vi "Na-DAS_and_MAGIC_Pressures.vi"() -> (0 "DAQ Error":errorcluster)   [LabVIEW 2017]
doc: "Use this plug-in with the Nathan 7609 data acquisition system"
uses:
  MAGIC_Pressures/ctls/Cmd.ctl
  Globals/Meas_global.vi
  PWA/PWAtasksGLOBAL.vi
  Globals/Extra_Commands_Global.vi
  Globals/Dynamic_call_global.ph.vi
  Globals/Trav_pos_global.vi
panel:
  in  "Board 2 COM port":refnum<visa-resource-name>="COM31"
  in  "Pressure data rate (Hz)":u8(ring)=17 items=["1", "2", "4", "5", "8", "10", "16", "20", "25", "32", "40", "50", "64", "80", "100", "125", "160", "200", "250", "320", "400", "500", "625", "800", "1000"]
  in  "Board 1 COM port":refnum<visa-resource-name>="COM30"
  in  "Minimum timeout (ms)":u32=15000
  in  "Input voltage range (V)":u8(ring)=1 items=["-5... +5 V", "-10... +10 V"]
  out "Config read-back ok":bool
  out "Overruns":u32
  # "PN 25/11/2014, 19/12/2014, 15/02/2015 (channels in any order), 17/08/2015 (stop ack mod), 23/08/2015 (timeout mod for SW vs HW triggering), 03/09/2017 (rising and falling edge options for HW triggering)"
  # "Do not close this window between blocks"
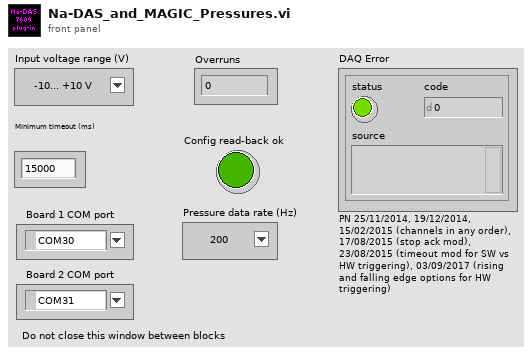
[diagram p1: front panel]
types:
  T1 = typedef "Ch_and_Spans.ctl" = cluster{"Sync Delay (ms)":dbl, "Ch No":i16, "Var name":string, "Use Latest Calib":bool, "Device ID":string}
  T2 = typedef "LDA_Setup.ctl" = cluster{"dimensions":enum16{"1D", "2D"}, "Analogue Freq Multiplier":dbl}
  T3 = typedef "Traverse_cluster.ctl" = cluster{"Start X":sgl, "Start Y":sgl, "Start Z":sgl, "End X":sgl, "End Y":sgl, "End Z":sgl, "No. of pts.":i32, "Spacing":T4, "Filename":path, "Tunnel Speed":dbl, "Averaging time (min)":dbl, "Extra Commands":string, "Carrier_1 Q (l/min)":dbl, "Carrier_2 Q (l/min)":dbl, "Trace Gas Concentration (%)":dbl, "Specific Arguments":string, "Comments":string, "Row No":i32, "Row Type Selector":T5, "Completion time":string, "Row Duration (mins)":dbl, "No. of Valid pts.":i32, "Meas Setup File":string}
  T4 = typedef "Spacing.ctl" = enum16{"Linear", "Log", "Gauss", "Specified", "N/A"}
  T5 = typedef "Multi_run_mode.ctl" = enum16{"Move Traverse Only", "Set Tunnel Speed Only", "Set Source Only", "Set Measurement Conditions", "Single Measurement", "Vertical Profile", "Lateral Profile", "Longitudinal Profile", "Explore Volume", "Multi-Axis Profile", "Auto Calibrate", "Meas Fast FID Bkgnd", "Check Beam Power", "Scanning Valve Measurement", "Run VI Named:", "Set ADAM Ch", "Wait (minutes)", "Send Message", "Synchronize With:", "Fall Back to this Row", "Turn Off Row Repeating", "Blank Row", "Traverse 3D Volume"}
  T6 = typedef "Trigger_Mode.ctl" = enum16{"Free Running", "Start on Trigger", "Trigger Every Block", "Trigger Every Sample"}
  T7 = typedef "Cmd.ctl" = string
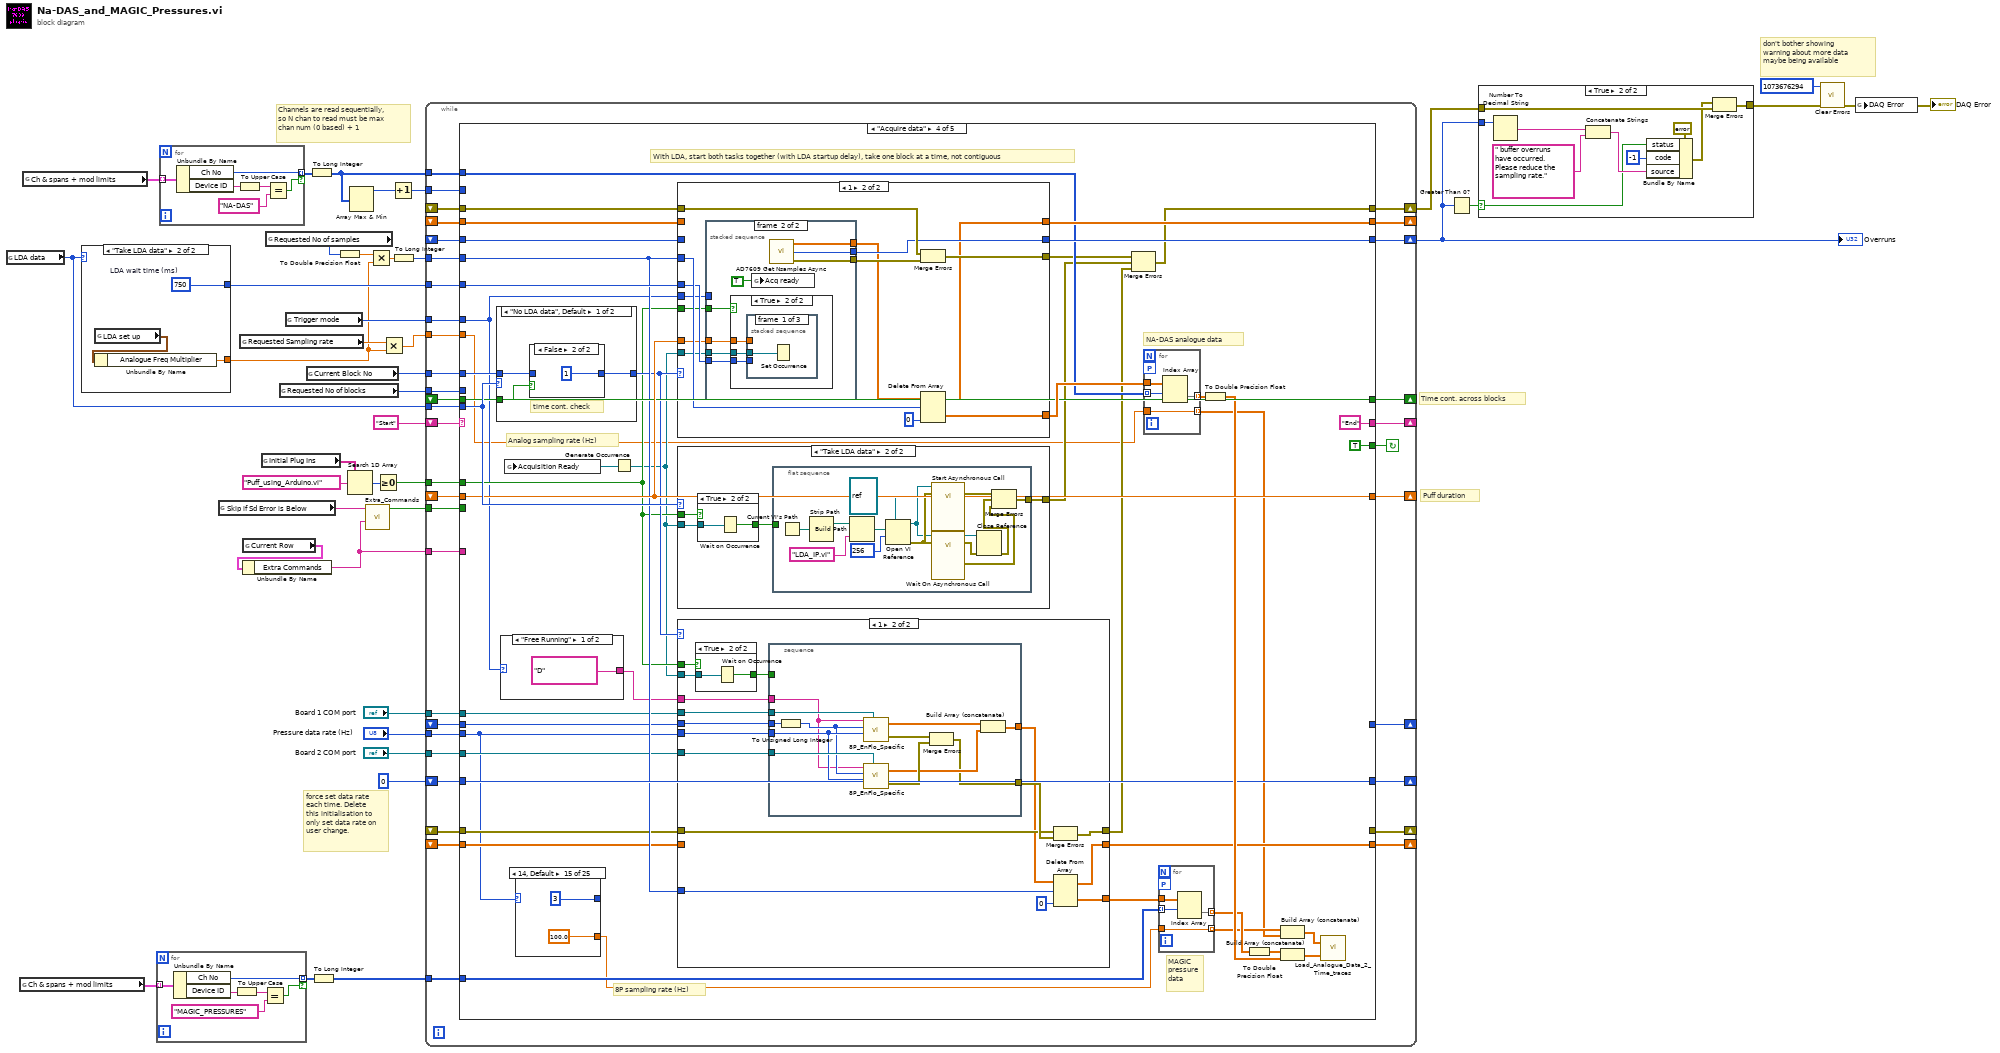
[diagram p0: block diagram]
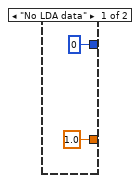
[diagram p2: hidden frame]
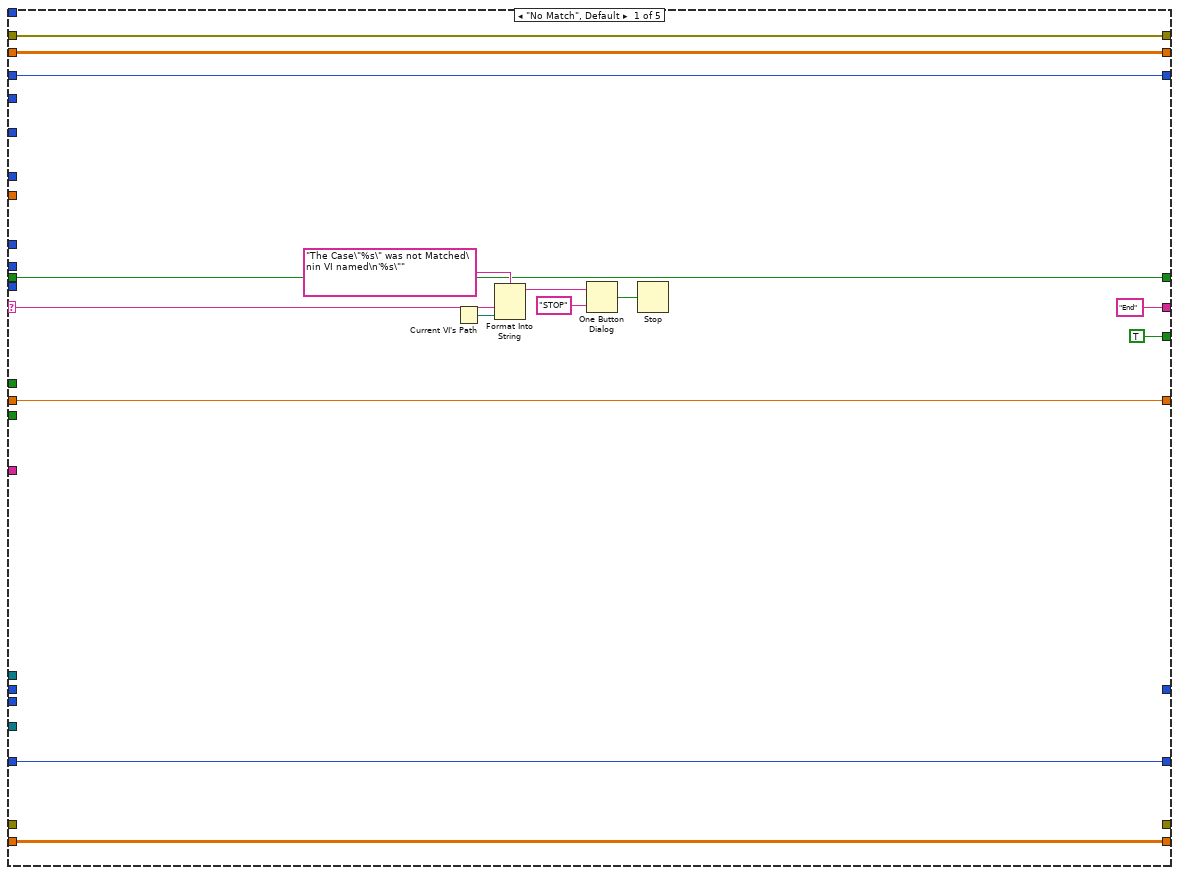
[diagram p3: hidden frame]
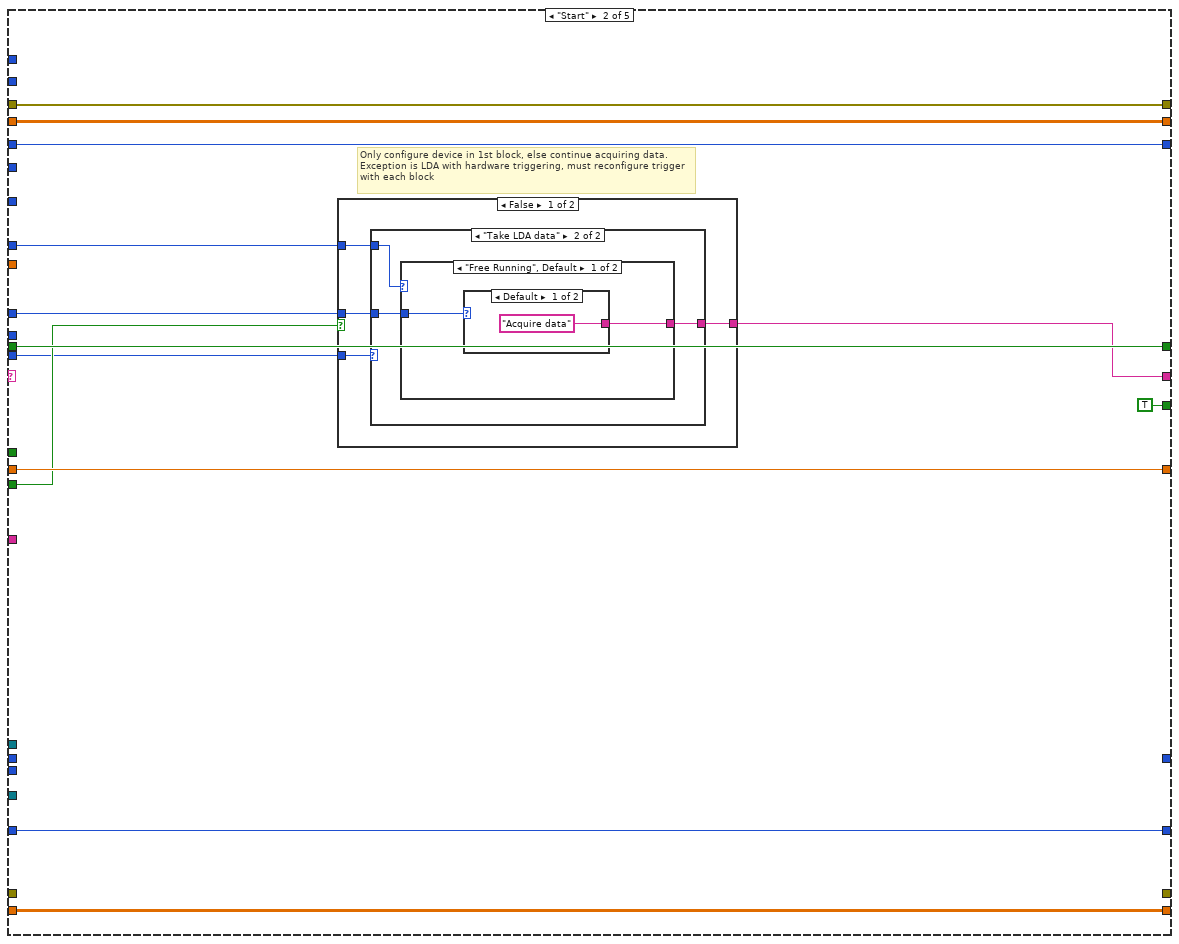
[diagram p4: hidden frame]
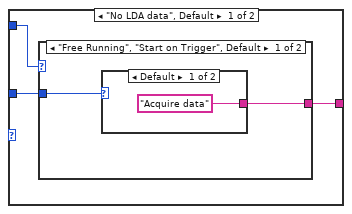
[diagram p5: hidden frame]
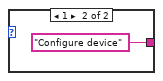
[diagram p6: hidden frame]
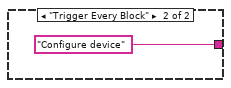
[diagram p7: hidden frame]
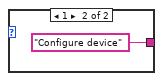
[diagram p8: hidden frame]
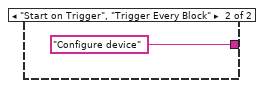
[diagram p9: hidden frame]
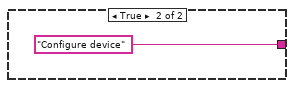
[diagram p10: hidden frame]
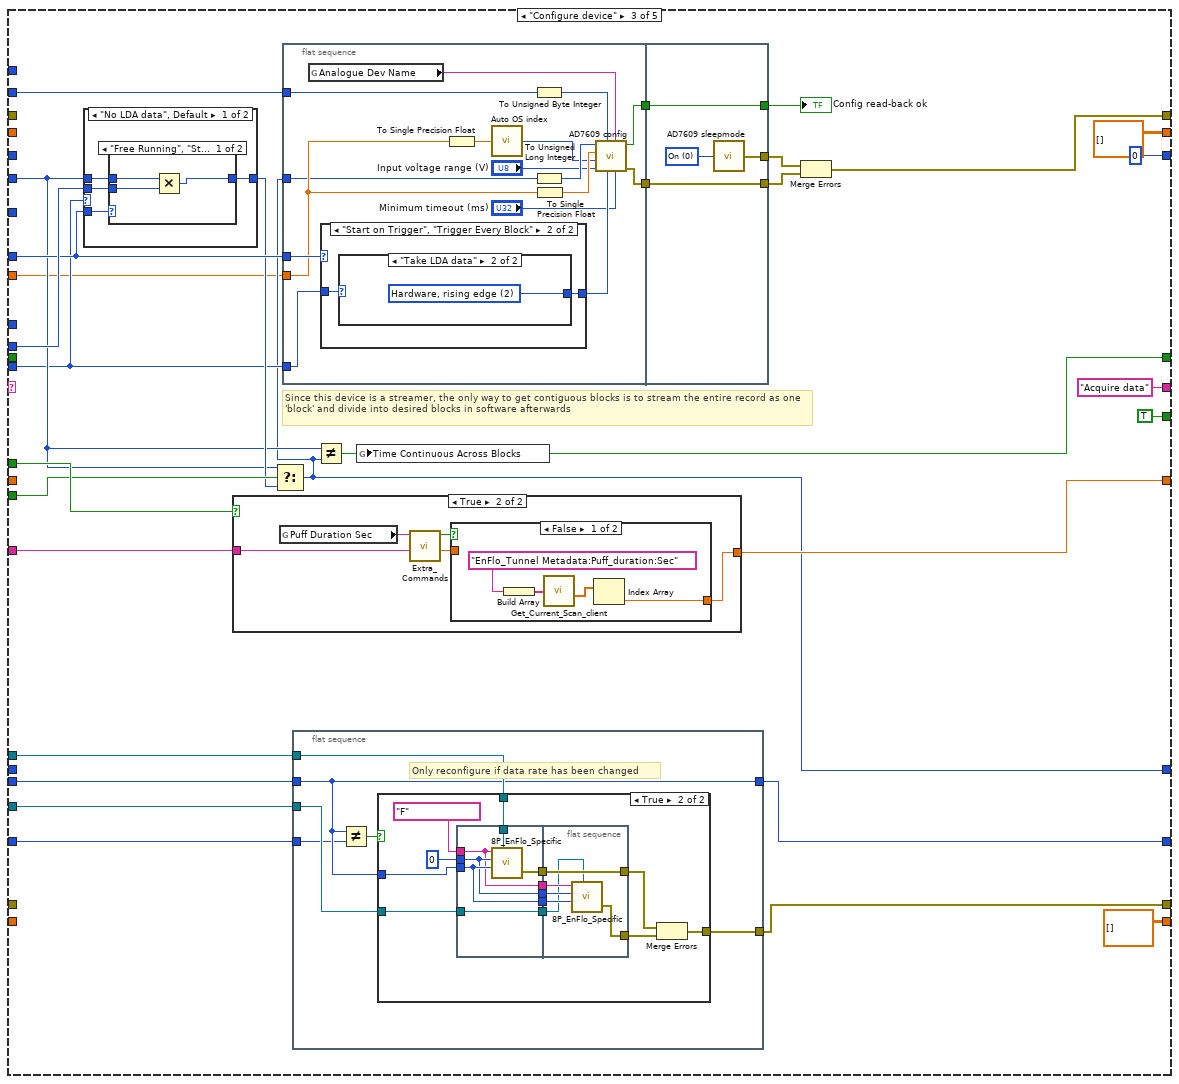
[diagram p11: hidden frame]
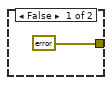
[diagram p12: hidden frame]
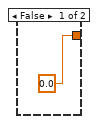
[diagram p13: hidden frame]
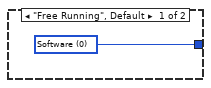
[diagram p17: hidden frame]
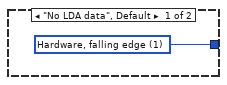
[diagram p18: hidden frame]
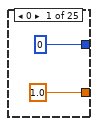
[diagram p19: hidden frame]
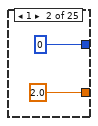
[diagram p20: hidden frame]
diagram:
  # "force set data rate each time. Delete this initialisation to only set data rate on user change."
  # "don't bother showing warning about more data maybe being available"
  # "Time cont. across blocks"
  # "Puff duration"
  # "Channels are read sequentially, so N chan to read must be max chan num (0 based) + 1"
  n1 = global read "Meas_global.vi" "LDA data"() -> (w34:enum16{"No LDA data", "Take LDA data"})
  n2 = global read "Meas_global.vi" "Ch & spans + mod limits"() -> (w3:T1[])
  n3 = global read "Meas_global.vi" "Ch & spans + mod limits"() -> (w20:T1[])
  n4 = case shown="\"Take LDA data\"" w34 {
    tunnel: [1.0 ("Analogue Freq Multiplier") w43] -> w25
    tunnel: [u32 0 ("LDA wait time (ms)") w42] -> w29
    frame "No LDA data" {
    }
    frame "Take LDA data" {
      w42 = u32 750  # LDA wait time (ms)
      n5 = global read "Meas_global.vi" "LDA set up"() -> (w44:T2)
      n6 = Unbundle By Name(w44) -> ("Analogue Freq Multiplier"=w43:dbl)
    }
  }
  n7 = for {
    tunnel: w3 -> [w50] mode=indexing
    tunnel: [w49] -> w4 mode=indexing if=w45
    n8 = Unbundle By Name(w50) -> ("Ch No"=w49:i16, "Device ID"=w48:string)
    n9 = To Upper Case(1:w48) -> (0:w47:string)
    n10 = Equal?(x=w47, y="MAGIC_PRESSURES") -> (x = y?=w45:bool)
  }
  n11 = for {
    tunnel: w20 -> [w56] mode=indexing
    tunnel: [w55] -> w19 mode=indexing if=w51
    n12 = Unbundle By Name(w56) -> ("Ch No"=w55:i16, "Device ID"=w54:string)
    n13 = To Upper Case(1:w54) -> (0:w53:string)
    n14 = Equal?(x=w53, y="NA-DAS") -> (x = y?=w51:bool)
  }
  n15 = global read "Extra_Commands_Global.vi" "Skip if Sd Error is Below"() -> (w15:string)
  n16 = global read "Meas_global.vi" "Requested Sampling rate"() -> (w35:dbl)
  n17 = global read "Trav_pos_global.vi" "Current Row"() -> (w16:T3)
  n18 = Unbundle By Name(w16) -> ("Extra Commands"=w14:string)
  n19 = global read "Dynamic_call_global.ph.vi" "Initial Plug Ins"() -> (w31:string[])
  n20 = global read "Meas_global.vi" "Requested No of samples"() -> (w26:i32)
  n21 = global read "Meas_global.vi" "Requested No of blocks"() -> (w22:i32)
  n22 = global read "Meas_global.vi" "Trigger mode"() -> (w38:T6)
  n23 = global read "Meas_global.vi" "Current Block No"() -> (w37:i32)
  n24 = To Long Integer(number=w19) -> (32bit integer=w1:i32[])
  n25 = To Long Integer(number=w4) -> (32bit integer=w2:i32[])
  n26 = To Double Precision Float(number=w26) -> (double precision float=w24:dbl)
  n27 = Search 1D Array(1D array=w31, element="Puff_using_Arduino.vi") -> (index of element=w33:i32)  [unwired: 1 in]
  n28 = Array Max & Min(array=w1) -> (max value=w18:i32)  [unwired: 3 out]
  n29 = call "Extra_Commands.vi"("String to Search"=w14, "Command"=w15) -> ("Command Found"=w13:bool)  [unwired: 2 in, 3 out]
  n30 = Multiply(x=w24, y=w25) -> (x*y=w23:dbl)
  n31 = Greater Or Equal To 0?(x=w33) -> (x >= 0?=w30:bool)
  n32 = Multiply(x=w35, y=w25) -> (x*y=w36:dbl)
  n33 = Increment(x=w18) -> (x+1=w17:i32)
  n34 = To Long Integer(number=w23) -> (32bit integer=w21:i32)
  n35 = while {
    shift-left: "Start" -> [w93]
    shift-right: [w79] -> _
    tunnel: w36 -> [w92]
    tunnel: w21 -> [w91]
    tunnel: w37 -> [w90]
    tunnel: w38 -> [w88]
    tunnel: w34 -> [w87]
    tunnel: w22 -> [w86]
    shift-right: [w84] -> w28
    shift-left: _ -> [w85]
    shift-right: [w83] -> _
    shift-left: _ -> [w82]
    shift-right: [w81] -> w11
    shift-left: _ -> [w80]
    tunnel: w29 -> [w78]
    tunnel: w30 -> [w77]
    shift-right: [w76] -> _
    shift-left: _ -> [w75]
    tunnel: w17 -> [w74]
    tunnel: w14 -> [w73]
    tunnel: w13 -> [w72]
    shift-right: [w71] -> _
    shift-left: _ -> [w70]
    tunnel: "Board 1 COM port" -> [w69]
    tunnel: "Pressure data rate (Hz)" -> [w68]
    tunnel: "Board 2 COM port" -> [w67]
    shift-right: [w65] -> _
    shift-left: u8 0 ("Pressure data rate (Hz)") -> [w66]
    shift-right: [w64] -> _
    shift-left: _ -> [w61]
    shift-right: [w62] -> _
    shift-left: _ -> [w63]
    shift-right: [w60] -> _
    shift-left: _ -> [w59]
    tunnel: w2 -> [w58]
    tunnel: w1 -> [w57]
    stop <- w89 continue-if-true
    n36 = case shown="\"Acquire data\"" w93 {
      selector: w93 -> [w101 _ _ _ _]
      tunnel: ["End" w111 "Acquire data" ("f") "End" "End" ("f")] -> w79
      tunnel: w92 -> [_ _ w143 w252 _]
      tunnel: w91 -> [_ _ w154 w272 _]
      tunnel: w90 -> [_ w114 _ w286 w467]
      tunnel: [TRUE TRUE TRUE TRUE FALSE] -> w89
      tunnel: w88 -> [_ w113 w161 w258 _]
      tunnel: w87 -> [_ w112 w152 w284 _]
      tunnel: w86 -> [_ _ w170 _ w468]
      tunnel: w85 -> [w100 w120 _ w291 w465]
      tunnel: [w100 w120 w171 w276 w464] -> w84
      tunnel: [w99 w119 sgl[][] [] ("Channel volts") w287 w463] -> w83
      tunnel: w82 -> [w99 w119 _ w288 w463]
      tunnel: [w98 w118 u32 0 ("Overruns") w290 w462] -> w81
      tunnel: w80 -> [w98 w118 _ w289 w462]
      tunnel: w78 -> [_ _ _ w285 _]
      tunnel: w77 -> [_ _ w160 w261 _]
      tunnel: [w97 w117 w159 w283 w461] -> w76
      tunnel: w75 -> [w97 w117 _ w283 w461]
      tunnel: w57 -> [_ _ _ w281 _]
      tunnel: w74 -> [_ _ w158 _ _]
      tunnel: w73 -> [_ _ w157 _ _]
      tunnel: w72 -> [_ w115 w156 _ _]
      tunnel: [w96 w116 w153 w279 w460] -> w71
      tunnel: w70 -> [w96 w116 _ w279 w460]
      tunnel: w69 -> [_ _ w151 w268 _]
      tunnel: w68 -> [_ _ w149 w251 _]
      tunnel: w67 -> [_ _ w150 w269 _]
      tunnel: w66 -> [w95 w110 w148 w273 w459]
      tunnel: [w95 w110 w147 w273 w459] -> w65
      tunnel: [_ _ w146 _ _] -> w64
      tunnel: w63 -> [_ _ _ w270 _]
      tunnel: [_ _ w145 _ _] -> w62
      tunnel: w61 -> [_ _ _ w267 _]
      tunnel: [w94 w109 sgl[][] [] ("Channel volts") w266 w458] -> w60
      tunnel: w59 -> [w94 w109 _ w263 w458]
      tunnel: w58 -> [_ _ _ w253 _]
      frame "No Match", Default {
        n37 = Current VI's Path() -> (path=w104:path)
        n38 = Format Into String(format string="The Case\"%s\" was not Matched\nin VI named\n'%s\"" ("Format String"), w101, w104) -> (resulting string=w107:string)  [unwired: 2 in, 1 out]
        n39 = One Button Dialog(message=w107, button name ("OK")="STOP") -> (true=w105:bool)
        n40 = Stop(stop? (T)=w105) -> ()
      }
      frame "Start" {
        # "Only configure device in 1st block, else continue acquiring data. Exception is LDA with hardware triggering, must reconfigure trigger with each block"
        n41 = case shown="False" w115 {
          tunnel: w114 -> [w125 _]
          tunnel: [w124 "Configure device" ("f")] -> w111
          tunnel: w112 -> [w123 _]
          tunnel: w113 -> [w122 _]
          frame False {
            n42 = case shown="\"Take LDA data\"" w123 {
              tunnel: w125 -> [w128 w134]
              tunnel: [w127 w135] -> w124
              tunnel: w122 -> [w126 w136]
              frame "No LDA data", Default {
                n43 = case shown="\"Free Running\", \"Start on Trigger\", Default" w126 {
                  tunnel: w128 -> [w130 _]
                  tunnel: [w129 "Configure device" ("f")] -> w127
                  frame "Free Running", "Start on Trigger", Default {
                    n44 = case shown="Default" w130 {
                      tunnel: ["Acquire data" ("f") "Configure device" ("f")] -> w129
                      frame Default {
                      }
                      frame 1 {
                      }
                    }
                  }
                  frame "Trigger Every Block" {
                  }
                }
              }
              frame "Take LDA data" {
                n45 = case shown="\"Free Running\", Default" w136 {
                  tunnel: [w138 "Configure device" ("f")] -> w135
                  tunnel: w134 -> [w137 _]
                  frame "Free Running", Default {
                    n46 = case shown="Default" w137 {
                      tunnel: ["Acquire data" ("f") "Configure device" ("f")] -> w138
                      frame Default {
                      }
                      frame 1 {
                      }
                    }
                  }
                  frame "Start on Trigger", "Trigger Every Block" {
                  }
                }
              }
            }
          }
          frame True {
          }
        }
      }
      frame "Configure device" {
        # "Since this device is a streamer, the only way to get contiguous blocks is to stream the entire record as one 'block' and divide into desired blocks in software afterwards"
        n47 = case shown="\"No LDA data\", Default" w152 {
          tunnel: [w217 w224] -> w155
          tunnel: w154 -> [w219 w224]
          tunnel: w170 -> [w218 _]
          tunnel: w161 -> [w216 _]
          frame "No LDA data", Default {
            n48 = case shown="\"Free Running\", \"Start on Trigger\"" w216 {
              tunnel: w219 -> [w222 w223]
              tunnel: w218 -> [w221 _]
              tunnel: [w220 w223] -> w217
              frame "Free Running", "Start on Trigger" {
                n49 = Multiply(x=w222, y=w221) -> (x*y=w220:i32)
              }
              frame "Trigger Every Block", Default {
              }
            }
          }
          frame "Take LDA data" {
          }
        }
        n50 = case shown="True" w160 {
          tunnel: [0.0 w210] -> w159
          tunnel: w157 -> [_ w206]
          frame False {
          }
          frame True {
            n51 = global read "Extra_Commands_Global.vi" "Puff Duration Sec"() -> (w209:string)
            n52 = call "Extra_Commands.vi"("String to Search"=w206, "Command"=w209) -> ("Numeric Value"=w207:dbl, "Command Found"=w208:bool)  [unwired: 2 in, 2 out]
            n53 = case shown="False" w208 {
              tunnel: [w211 w215] -> w210
              tunnel: w207 -> [_ w215]
              frame False {
                n54 = Build Array("EnFlo_Tunnel Metadata:Puff_duration:Sec") -> (w213:string[])
                n55 = call "Get_Current_Scan_client.vi"("ADAM Ch Names"=w213) -> ("Numerical Values"=w214:dbl[])  [unwired: 1 in, 2 out]
                n56 = Index Array(array=w214) -> (element=w211:dbl)  [unwired: 1 in]
              }
              frame True {
              }
            }
          }
        }
        n57 = Select(t=w154, s=w156, f=w155) -> (s? t:f=w146:i32)
        n58 = flat-sequence {
          tunnel: w146 -> [w225]
          tunnel: w143 -> [w231]
          tunnel: w161 -> [w240]
          tunnel: [w234] -> w169
          tunnel: [w233] -> w168
          tunnel: w158 -> [w228]
          tunnel: w152 -> [w226]
          tunnel: [w248] -> w165
          tunnel: w169 -> [w248]
          tunnel: [w247] -> w167
          tunnel: w168 -> [w247]
          tunnel: [w246] -> w166
          frame #0 {
            n59 = global read "PWAtasksGLOBAL.vi" "Analogue Dev Name"() -> (w239:string)
            n60 = case shown="\"Start on Trigger\", \"Trigger Every Block\"" w240 {
              tunnel: [w241 w243] -> w236
              tunnel: w226 -> [_ w242]
              frame "Free Running", Default {
                w241 = u8 0 items=["Software", "Hardware, falling edge", "Hardware, rising edge"] ("Triggering mode")
              }
              frame "Start on Trigger", "Trigger Every Block" {
                n61 = case shown="\"Take LDA data\"" w242 {
                  tunnel: [w244 w245] -> w243
                  frame "No LDA data", Default {
                    w244 = u8 1 items=["Software", "Hardware, falling edge", "Hardware, rising edge"] ("Triggering mode")
                  }
                  frame "Take LDA data" {
                    w245 = u8 2 items=["Software", "Hardware, falling edge", "Hardware, rising edge"] ("Triggering mode")
                  }
                }
              }
            }
            n62 = To Single Precision Float(number=w231) -> (single precision float=w229:sgl)
            n63 = call "Auto OS index.vi"("Sampling rate"=w229) -> ("OS index"=w230:u8)
            n64 = To Unsigned Byte Integer(number=w228) -> (unsigned 8bit integer=w235:u8)
            n65 = To Unsigned Long Integer(number=w225) -> (unsigned 32bit integer=w238:u32)
            n66 = To Single Precision Float(number=w231) -> (single precision float=w237:sgl)
            n67 = call "AD7609 config.vi"("Timeout for software trig. mode (ms)"="Minimum timeout (ms)", "Device serial port"=w239, "Triggering mode"=w236, "N channels to read"=w235, "Input voltage range (V)"="Input voltage range (V)", "Oversampling ratio"=w230, "Sampling rate (Hz)"=w237, "Number of samples"=w238) -> ("Config error out"=w233:errorcluster, "Config read-back ok"=w234:bool)  [unwired: 2 in]
          }
          frame #1 {
            w249 = u8 0 items=["On", "Standby", "Shutdown"] ("Sleep state")
            n68 = call "AD7609 sleepmode.vi"("Sleep state"=w249) -> ("Sleep error out"=w246:errorcluster)
          }
        }
        n69 = flat-sequence {
          tunnel: [w178] -> w145
          tunnel: w151 -> [w177]
          tunnel: w150 -> [w176]
          tunnel: w149 -> [w174]
          tunnel: [w174] -> w147
          tunnel: w148 -> [w173]
          frame #0 {
            # "Only reconfigure if data rate has been changed"
            n70 = Not Equal?(x=w174, y=w173) -> (x != y?=w175:bool)
            n71 = case shown="True" w175 {
              tunnel: [errorcluster {"status"=FALSE, "code"=0, "source"=""} ("error IO") w191] -> w178
              tunnel: w177 -> [_ w190]
              tunnel: w176 -> [_ w180]
              tunnel: w174 -> [_ w187]
              frame False {
              }
              frame True {
                n72 = flat-sequence {
                  tunnel: w190 -> [w194]
                  tunnel: T7 "F" ("Command") -> [w195]
                  tunnel: u32 0 ("N samples") -> [w196]
                  tunnel: w187 -> [w197]
                  tunnel: [w198] -> w185
                  tunnel: [w197] -> w184
                  tunnel: [w196] -> w183
                  tunnel: [w195] -> w182
                  tunnel: [w193] -> w181
                  tunnel: w180 -> [w193]
                  tunnel: [w204] -> w192
                  tunnel: [w200] -> w186
                  tunnel: w181 -> [w199]
                  tunnel: w182 -> [w201]
                  tunnel: w183 -> [w202]
                  tunnel: w184 -> [w203]
                  tunnel: w185 -> [w204]
                  frame #0 {
                    n73 = call "8P_EnFlo_Specific.vi"("COM port"=w194, "Data rate (Hz)"=w197, "N samples"=w196, "Command"=w195) -> ("Error"=w198:errorcluster)  [unwired: 2 in, 1 out]
                  }
                  frame #1 {
                    n74 = call "8P_EnFlo_Specific.vi"("COM port"=w199, "Data rate (Hz)"=w203, "N samples"=w202, "Command"=w201) -> ("Error"=w200:errorcluster)  [unwired: 2 in, 1 out]
                  }
                }
                n75 = Merge Errors(w192, w186) -> (w191:errorcluster)
              }
            }
          }
        }
        n76 = Not Equal?(x=w154, y=w146) -> (x != y?=w153:bool)
        n77 = global write "Meas_global.vi" "Time Continuous Across Blocks"(w153) -> ()
        n78 = Merge Errors(w166, w167) -> (w171:errorcluster)
        "Config read-back ok" <- w165
      }
      frame "Acquire data" {
        # "Analog sampling rate (Hz)"
        # "8P sampling rate (Hz)"
        # "MAGIC\npressure\ndata"
        # "NA-DAS analogue data"
        # "With LDA, start both tasks together (with LDA startup delay), take one block at a time, not contiguous"
        n79 = case shown="\"No LDA data\", Default" w284 {
          tunnel: w286 -> [w414 _]
          tunnel: [w415 1 ("Current Block No")] -> w271
          tunnel: w279 -> [w413 _]
          frame "No LDA data", Default {
            # "time cont. check"
            n80 = case shown="False" w413 {
              tunnel: [w416 1 ("Current Block No")] -> w415
              tunnel: w414 -> [w416 _]
              frame True {
              }
              frame False {
              }
            }
          }
          frame "Take LDA data" {
          }
        }
        n81 = case shown="\"Free Running\"" w258 {
          tunnel: [T7 "D" ("Combo Box") T7 "T" ("Combo Box")] -> w257
          frame "Free Running" {
          }
          frame Default {
          }
        }
        n82 = case shown="14, Default" w251 {
          tunnel: [1.0 2.0 4.0 5.0 8.0 10.0 16.0 20.0 25.0 32.0 40.0 50.0 64.0 80.0 100.0 125.0 160.0 200.0 250.0 320.0 400.0 500.0 625.0 800.0 1000.0] -> w250
          tunnel: [u8 0 u8 0 u8 0 u8 0 u8 0 u8 0 u8 0 u8 0 u8 1 u8 1 u8 1 u8 2 u8 2 u8 2 u8 3 u8 3 u8 3 u8 4 u8 4 u8 4 u8 5 u8 5 u8 6 u8 6 u8 6] -> _
          frame 0 {
          }
          frame 1 {
          }
          frame 2 {
          }
          frame 3 {
          }
          frame 4 {
          }
          frame 5 {
          }
          frame 6 {
          }
          frame 7 {
          }
          frame 8 {
          }
          frame 9 {
          }
          frame 10 {
          }
          frame 11 {
          }
          frame 12 {
          }
          frame 13 {
          }
          frame 14, Default {
          }
          frame 15 {
          }
          frame 16 {
          }
          frame 17 {
          }
          frame 18 {
          }
          frame 19 {
          }
          frame 20 {
          }
          frame 21 {
          }
          frame 22 {
          }
          frame 23 {
          }
          frame 24 {
          }
        }
        n83 = Generate Occurrence() -> (w260:refnum<k4>)
        n84 = global write "Meas_global.vi" "Acquisition Ready"(w260) -> ()
        n85 = case shown="1" w271 {
          tunnel: w291 -> [w420 w438]
          tunnel: [w420 w437] -> w278
          tunnel: [w421 w436] -> w290
          tunnel: [w423 w433] -> w287
          tunnel: w272 -> [w422 w434]
          tunnel: w288 -> [w424 _]
          tunnel: w289 -> [w421 _]
          tunnel: [w419 w431] -> w282
          tunnel: w285 -> [_ w430]
          tunnel: w260 -> [_ w429]
          tunnel: w261 -> [_ w428]
          tunnel: w283 -> [_ w427]
          tunnel: w258 -> [_ w426]
          frame Default {
            # "First block gets ALL samples (N_blocks * samples per block). Output one block of samples and keep remainder for next block cycle."
            n86 = Delete From Array(array=w424, length=w422, index (col)=0 ("disabled index (col)")) -> (deleted portion=w419:sgl[][], array with subset deleted=w423:sgl[][])  [unwired: 1 in]
          }
          frame 1 {
            n87 = stacked-sequence {
              tunnel: [_ w449] -> w436
              tunnel: [_ w448] -> w435
              tunnel: [_ w447] -> w439
              tunnel: w429 -> [_ w446]
              tunnel: w430 -> [w441 w445]
              tunnel: w428 -> [_ w444]
              tunnel: w427 -> [_ w443]
              tunnel: w426 -> [w440 _]
              frame #0 {
                n88 = case shown="\"Free Running\"" w440 {
                  tunnel: w441 -> [w442 _]
                  frame "Free Running" {
                    n89 = Wait (ms)(milliseconds to wait=w442) -> ()  [unwired: 1 out]
                  }
                  frame Default {
                  }
                }
              }
              frame #1 {
                n90 = case shown="True" w444 {
                  tunnel: w446 -> [w451 w454]
                  tunnel: w443 -> [_ w453]
                  tunnel: w445 -> [_ w452]
                  frame False {
                    n91 = Set Occurrence(w451) -> ()
                  }
                  frame True {
                    n92 = stacked-sequence {
                      tunnel: w454 -> [w455 _ _]
                      tunnel: w453 -> [_ _ w457]
                      tunnel: w452 -> [_ w456 _]
                      frame #0 {
                        n93 = Set Occurrence(w455) -> ()
                      }
                      frame #1 {
                        n94 = Wait (ms)(milliseconds to wait=w456) -> ()  [unwired: 1 out]
                      }
                      frame #2 {
                        n95 = call "Puff_using_Arduino_oneshot.vi"("Puff_duration:Sec"=w457) -> ()  [unwired: 7 in]
                      }
                    }
                  }
                }
                n96 = global write "Meas_global.vi" "Acq ready"(TRUE ("Acq ready")) -> ()
                n97 = call "AD7609 Get Nsamples Async.vi"() -> ("Channel volts"=w448:sgl[][], "Overruns"=w449:u32, "Async error"=w447:errorcluster)  [unwired: 1 in]
              }
            }
            n98 = Merge Errors(w438, w439) -> (w437:errorcluster)
            n99 = Delete From Array(array=w435, length=w434, index (col)=0 ("disabled index (col)")) -> (deleted portion=w431:sgl[][], array with subset deleted=w433:sgl[][])  [unwired: 1 in]
          }
        }
        n100 = case shown="\"Take LDA data\"" w284 {
          tunnel: w261 -> [_ w392]
          tunnel: w260 -> [_ w394]
          tunnel: [errorcluster {"status"=FALSE, "code"=0, "source"=""} ("error IO") w393] -> w277
          frame "No LDA data", Default {
          }
          frame "Take LDA data" {
            n101 = case shown="True" w392 {
              tunnel: [FALSE ("timed out") w398] -> w395
              tunnel: w394 -> [_ w397]
              frame False {
              }
              frame True {
                n102 = Wait on Occurrence(2:w397) -> (0:w398:bool)  [unwired: 2 in]
              }
            }
            n103 = flat-sequence {
              tunnel: w395 -> [_]
              tunnel: [w400] -> w393
              frame #0 {
                n104 = Current VI's Path() -> (path=w410:path)
                n105 = Strip Path(path=w410) -> (stripped path=w409:path)  [unwired: 1 out]
                n106 = Build Path(base path=w409, name or relative path="LDA_IP.vi") -> (appended path=w411:path)
                n107 = Open VI Reference(type specifier VI Refnum (for type only)=refnum<vi> refnum, vi path=w411, options=256) -> (vi reference=w405:refnum<vi>, error out=w406:errorcluster)  [unwired: 3 in]
                n108 = call-by-ref "Start Asynchronous Call"(reference=w405, error in=w406) -> (error out=w402:errorcluster)  [unwired: 1 in, 2 out]
                n109 = call-by-ref "Wait On Asynchronous Call"(reference=w405, error in=w406) -> (reference out=w404:refnum<vi>, error out=w403:errorcluster, 0:"error out"=w399:errorcluster)  [unwired: 1 in]
                n110 = Close Reference(reference=w404, error in (no error)=w403) -> (error out=w401:errorcluster)
                n111 = Merge Errors(w402, w401, w399) -> (w400:errorcluster)
              }
            }
          }
        }
        n112 = case shown="1" w271 {
          tunnel: w270 -> [w351 w370]
          tunnel: [w351 w369] -> w262
          tunnel: [w353 w366] -> w266
          tunnel: w272 -> [w352 w367]
          tunnel: w263 -> [w354 _]
          tunnel: [w350 w364] -> w265
          tunnel: w268 -> [_ w363]
          tunnel: w269 -> [_ w362]
          tunnel: w251 -> [_ w361]
          tunnel: w267 -> [_ w360]
          tunnel: w261 -> [_ w358]
          tunnel: w260 -> [_ w357]
          tunnel: w257 -> [_ w356]
          frame Default {
            # "First block gets ALL samples (N_blocks * samples per block). Output one block of samples and keep remainder for next block cycle."
            n113 = Delete From Array(array=w354, length=w352, index (col)=0 ("disabled index (col)")) -> (deleted portion=w350:sgl[][], array with subset deleted=w353:sgl[][])  [unwired: 1 in]
          }
          frame 1 {
            n114 = case shown="True" w358 {
              tunnel: [FALSE ("timed out") w374] -> w359
              tunnel: w357 -> [_ w373]
              frame False {
              }
              frame True {
                n115 = Wait on Occurrence(2:w373) -> (0:w374:bool)  [unwired: 2 in]
              }
            }
            n116 = stacked-sequence {
              tunnel: [w378] -> w368
              tunnel: [w377] -> w371
              tunnel: w363 -> [w384]
              tunnel: w362 -> [w383]
              tunnel: w361 -> [w382]
              tunnel: w360 -> [w379]
              tunnel: w359 -> [_]
              tunnel: w356 -> [w375]
              frame #0 {
                n117 = To Unsigned Long Integer(number=w379) -> (unsigned 32bit integer=w376:u32)
                n118 = call "8P_EnFlo_Specific.vi"("COM port"=w384, "Data rate (Hz)"=w382, "N samples"=w376, "Command"=w375) -> ("Error"=w385:errorcluster, "All samples out"=w380:sgl[][])  [unwired: 2 in]
                n119 = call "8P_EnFlo_Specific.vi"("COM port"=w383, "Data rate (Hz)"=w382, "N samples"=w376, "Command"=w375) -> ("Error"=w386:errorcluster, "All samples out"=w381:sgl[][])  [unwired: 2 in]
                n120 = Merge Errors(w385, w386) -> (w377:errorcluster)
                n121 = Build Array (concatenate)(w380, w381) -> (w378:sgl[][])
              }
            }
            n122 = Merge Errors(w370, w371) -> (w369:errorcluster)
            n123 = Delete From Array(array=w368, length=w367, index (col)=0 ("disabled index (col)")) -> (deleted portion=w364:sgl[][], array with subset deleted=w366:sgl[][])  [unwired: 1 in]
          }
        }
        n124 = Merge Errors(w278, w277, w262) -> (w276:errorcluster)
        n125 = for {
          tunnel: w281 -> [w389] mode=indexing
          tunnel: [w388] -> w280 mode=indexing
          workers-P: _ -> [_]
          tunnel: w282 -> [w390]
          tunnel: [w387] -> w255 mode=indexing
          tunnel: w252 -> [w387]
          n126 = Index Array(array=w390, index (row)=w389) -> (element=w388:sgl[])  [unwired: 1 in]
        }
        n127 = for {
          tunnel: w253 -> [w348] mode=indexing
          tunnel: [w347] -> w264 mode=indexing
          workers-P: _ -> [_]
          tunnel: w265 -> [w349]
          tunnel: [w346] -> w256 mode=indexing
          tunnel: w250 -> [w346]
          n128 = Index Array(array=w349, index (row)=w348) -> (element=w347:sgl[])  [unwired: 1 in]
        }
        n129 = To Double Precision Float(number=w280) -> (double precision float=w274:dbl[][])
        n130 = To Double Precision Float(number=w264) -> (double precision float=w275:dbl[][])
        n131 = Build Array (concatenate)(w256, w255) -> (w254:dbl[])
        n132 = Build Array (concatenate)(w275, w274) -> (w259:dbl[][])
        n133 = call "Load_Analogue_Data_2_Time_traces.vi"("Voltage Array"=w259, "Sampling Rate (Hz)"=w254) -> ()  [unwired: 1 in]
      }
      frame "End" {
        n134 = Equal?(x=w467, y=w468) -> (x = y?=w466:bool)
        n135 = case shown="True" w466 {
          tunnel: w465 -> [w472 w474]
          tunnel: [w472 w473] -> w464
          frame False {
          }
          frame True {
            w476 = u8 1 items=["On", "Standby", "Shutdown"] ("Sleep state")
            n136 = call "AD7609 sleepmode.vi"("Sleep state"=w476) -> ("Sleep error out"=w475:errorcluster)
            n137 = Merge Errors(w474, w475) -> (w473:errorcluster)
          }
        }
        n138 = global write "Meas_global.vi" "Acq ready"(FALSE ("Acq ready")) -> ()
      }
    }
  }
  "Overruns" <- w11
  n139 = Greater Than 0?(x=w11) -> (x > 0?=w12:bool)
  n140 = case shown="True" w12 {
    selector: w12 -> [_ w479]
    tunnel: w28 -> [w477 w486]
    tunnel: [w477 w487] -> w27
    tunnel: w11 -> [_ w485]
    frame False {
    }
    frame True {
      n141 = Number To Decimal String(number=w485) -> (decimal integer string=w483:string)  [unwired: 1 in]
      n142 = Concatenate Strings(w483, " buffer overruns have occurred. Please reduce the sampling rate.") -> (w481:string)
      n143 = Bundle By Name(cluster=errorcluster {"status"=FALSE, "code"=0, "source"=""} ("error IO"), "status"=w479, "code"=-1, "source"=w481) -> (w478:errorcluster)
      n144 = Merge Errors(w478, w486) -> (w487:errorcluster)
    }
  }
  n145 = call <vilib>:"Clear Errors.vi"("error in (no error)"=w27, "specific error code to clear (0: all)"=1073676294) -> ("error out"=w10:errorcluster)  [unwired: 4 in, 1 out]
  "DAQ Error" <- w10
  n146 = global write "Meas_global.vi" "DAQ Error"(w10) -> ()
